vi "Load Into Sub Panel.vi"(8 "error in (no error)":cluster{"状态":bool, "代码":i32, "源":string} caption="错误输入（无错误）", 10 "用于子面板的VI":refnum<vi>, 11 "气冷系统应用程序输入":refnum<class "Air Cooler Application.lvclass">) -> (0 "error out":cluster{"状态":bool, "代码":i32, "源":string} caption="错误输出", 3 "气冷系统应用程序输出":refnum<class "Air Cooler Application.lvclass">)   [LabVIEW 2015, in "Air Cooler Application.lvlib" / "Air Cooler Application.lvclass"]
uses:
  Air Cooler Application.lvclass
  Air Cooler Application.lvclass/Air Cooler Application.ctl
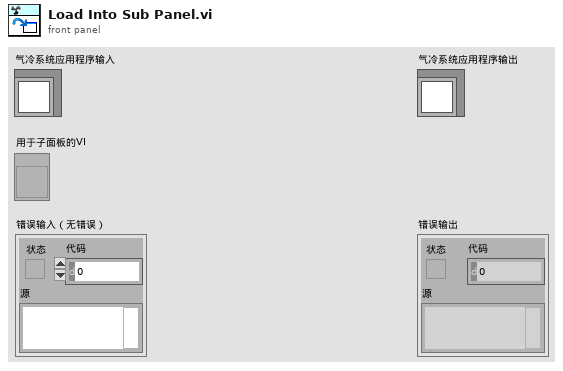
[diagram p1: front panel]
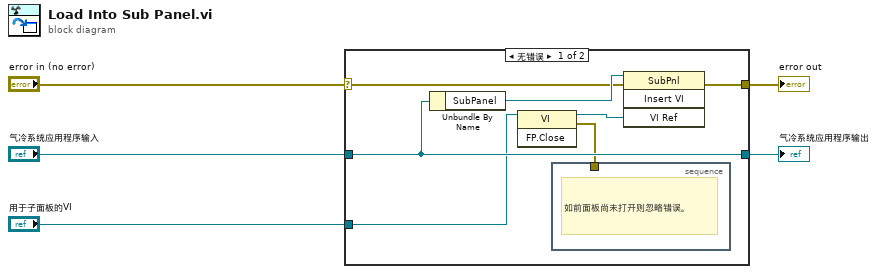
[diagram p0: block diagram]
diagram:
  n1 = case shown="无错误" "error in (no error)" {
    selector: "error in (no error)" -> [w10 w14]
    tunnel: [w9 w14] -> w4
    tunnel: [w12 w13] -> w2
    tunnel: "气冷系统应用程序输入" -> [w12 w13]
    tunnel: "用于子面板的VI" -> [w8 _]
    frame No Error {
      n2 = Unbundle By Name(w12) -> ("SubPanel"=w11:refnum<vi>)
      n3 = invoke class="VI" method="FP.Close"(reference=w8) -> (reference out=w7:refnum<vi>, error out=w6:errorcluster)  [unwired: 2 in, 1 out]
      n4 = stacked-sequence {
        tunnel: w6 -> [_]
        frame #0 {
          # "如前面板尚未打开则忽略错误。"
        }
      }
      n5 = invoke on="Invoke Node" class="SubPnl" method="Insert VI"(reference=w11, error in=w10, "VI Ref"=w7) -> (error out=w9:errorcluster)  [unwired: 1 in, 3 out]
    }
    frame Error {
    }
  }
  "error out" <- w4
  "气冷系统应用程序输出" <- w2
